vi "RSZVB Set Sweep Type.vi"(8 "error in (no error)":errorcluster {"code" format="%.0x"}, 9 "Sweep Type (0: Lin. Frequency)":i32(ring)=3 items=["Lin. Frequency", "Log. Frequency", "Segmented Frequency", "Power", "Time", "CW Mode", "Pulse", "Amplitude Imbalance Sweep", "Phase Imbalance Sweep"], 10 "Channel (1)":i32=1, 11 "VISA session":refnum<visa-resource-name>) -> (0 "error out":errorcluster {"code" format="%.0x"}, 3 "dup VISA session":refnum<visa-resource-name>)   [LabVIEW 2015]
doc: "This VI selects the sweep type, i.e. the sweep variable (frequency/power/time) and the position of the sweep points across the sweep range.\n\nRemote-control command(s):\n[SENSe<Ch>:]SWEep:TYPE LINear | LOGarithmic | SEGMent | POWer | CW | POINt | PULSe | IAMPlitude | IPHase"
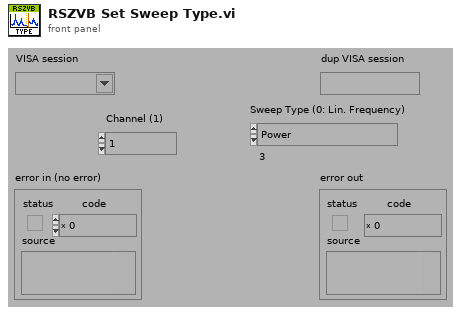
[diagram p1: front panel]
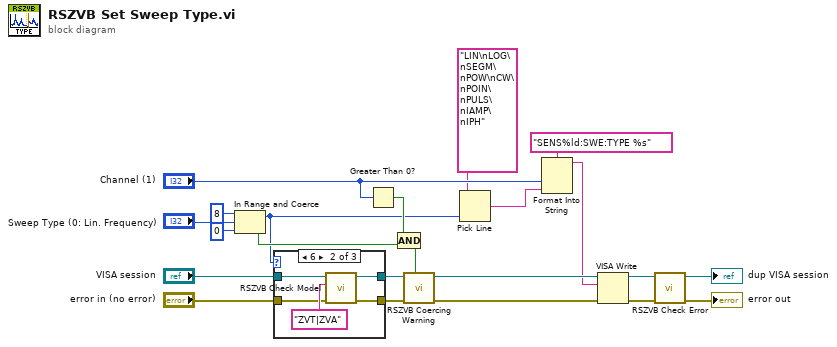
[diagram p0: block diagram]
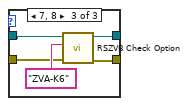
[diagram p3: hidden frame]
diagram:
  n1 = In Range and Coerce(upper limit=8, x="Sweep Type (0: Lin. Frequency)", lower limit=0) -> (coerced(x)=w1:i32, In Range?=w12:bool)
  n2 = case shown="6" w1 {
    tunnel: [w23 w28 w30] -> w5
    tunnel: [w24 w27 w31] -> w4
    tunnel: "VISA session" -> [w24 w26 w33]
    tunnel: "error in (no error)" -> [w23 w25 w32]
    frame 0, Default {
    }
    frame 6 {
      n3 = call "RSZVB Check Model.vi"("error in (no error)"=w25, "Model"="ZVT|ZVA" ("Options"), "VISA session"=w26) -> ("error out"=w28:errorcluster, "dup VISA session"=w27:refnum<visa-resource-name>)  [unwired: 7 in]
    }
    frame 7, 8 {
      n4 = call "RSZVB Check Option.vi"("error in (no error)"=w32, "Options"="ZVA-K6", "VISA session"=w33) -> ("error out"=w30:errorcluster, "dup VISA session"=w31:refnum<visa-resource-name>)  [unwired: 7 in]
    }
  }
  n5 = Greater Than 0?(x="Channel (1)") -> (x > 0?=w15:bool)
  n6 = Compound Arithmetic op=AND(w15, w12) -> (w17:bool)
  n7 = call "RSZVB Coercing Warning.vi"("In Range?"=w17, "error in (no error)"=w5, "VISA session"=w4) -> ("error out"=w20:errorcluster, "dup VISA session"=w21:refnum<visa-resource-name>)  [unwired: 7 in]
  n8 = Pick Line(multi-line string="LIN\nLOG\nSEGM\nPOW\nCW\nPOIN\nPULS\nIAMP\nIPH", line index=w1) -> (output string=w7:string)  [unwired: 1 in]
  n9 = Format Into String(format string="SENS%ld:SWE:TYPE %s", "Channel (1)", w7) -> (resulting string=w16:string)  [unwired: 2 in, 1 out]
  n10 = VISA Write(VISA resource name=w21, write buffer=w16, error in (no error)=w20) -> (VISA resource name out=w18:refnum<visa-resource-name>, error out=w19:errorcluster)  [unwired: 1 out]
  n11 = call "RSZVB Check Error.vi"("error in (no error)"=w19, "VISA session"=w18) -> ("error out"=→"error out":errorcluster, "dup VISA session"=→"dup VISA session":refnum<visa-resource-name>)  [unwired: 8 in]
